vi "Constants.vi"() -> ()   [LabVIEW 2019, in "WaveFormCustomDevice Shared.lvlib"]
doc: "Use this Global VI to access the GUIDs assigned to the page resources of the Custom Device."
uses:
  WaveFormCustomDevice Shared.lvlib
panel:
  in  "Tab Control":enum32{"GUIDS", "Constants", "Properties"}(tab)
  in  "WaveFormCustomDevice":string="1ce08059-5b27-4546-9e73-2f623b170946"
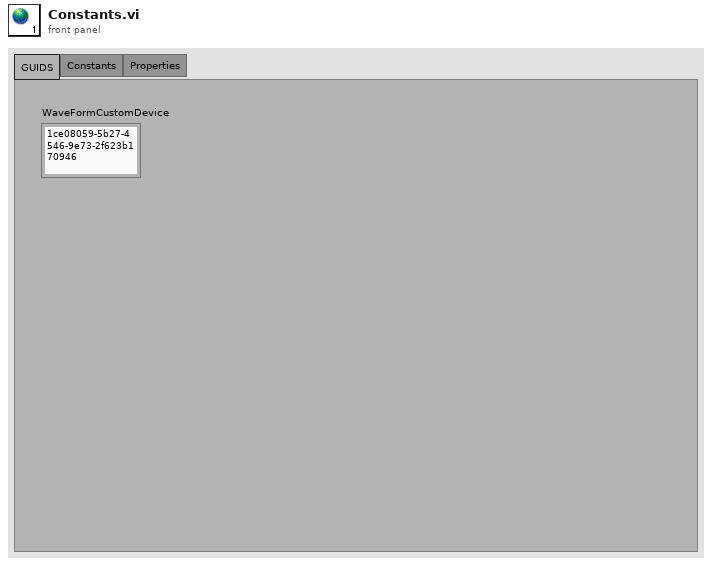
[diagram p1: front panel]
diagram:
